vi "HostPC.vi"() -> ()   [LabVIEW 2020]
doc: "Main VI on the host PC. It has an initializisation and an operational phase\n\nThe operational phase has two while loops. One input and one output loop that handle the in/output of the cRio."
uses:
  Status_cRio.ctl
  ElementDTD.lvlib
panel:
  in  "additonal Mass[g]":dbl
  out "Exp_id":i32
  out "Status":T1=enum."1_start_up"
  out "Loginname":string caption="Username"
  in  "OFF":bool
  out "Error PC":bool
  out "SuID":dbl caption="Subject ID" format="%#g"
  out "ImID":dbl caption="Impactor ID" format="%#g"
  in  "Start":bool
  in  "Subject Height[mm]":dbl
  in  "Inspect":bool
  in  "Mode selcection":enum16{"Normal", "Auto", "Manual"}(ring)
  out "Table Position":dbl
  in  "Registerkartenelement":enum32{"Normal", "Auto", "Manual", "Settings"}(tab)
  out "Out of bounds":bool
  in  "Impact Speed [m/s]":dbl
  out "Target Height [mm]":dbl
  in  "Tabel Input [mm]":dbl
  out "Normal Mode:":string
  in  "Table Inputs":dbl[](array[numeric])
  in  "Impact Speeds":dbl[](array[numeric])
  out "Auto Mode:":string
  out "No Data":bool
  out "Index":i32
  in  "Table Input [mm]":dbl
  in  "Carrier Input [mm]":dbl
  in  "Solenoids":bool
  in  "Magnets":bool
  out "Normal/Repair Mode:":string
  in  "Humidity":dbl
  in  "Data Export":bool
  in  "Dialog":bool
  in  "Repair":bool
  in  "Stopp":bool
  out "Name":string
  out "Error cRio":bool
  in  "Skip Cam":bool
  out "Carrier Height":dbl
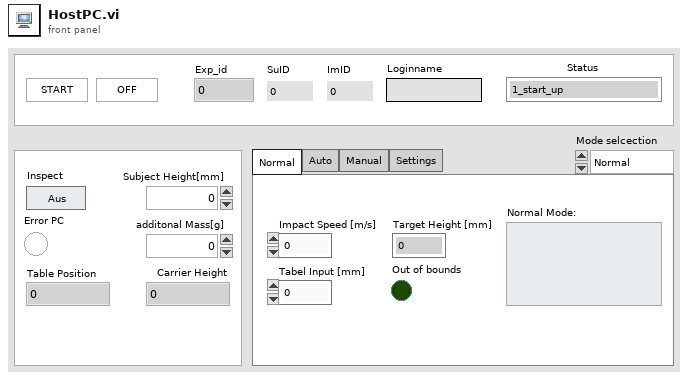
[diagram p1: front panel]
types:
  T1 = typedef "ElementDTD.lvlib/Status_cRio.ctl" = enum16{"0_Error", "1_start_up", "4_moving_to_position", "5_measure", "6_DataExport", "7_turnOff"}
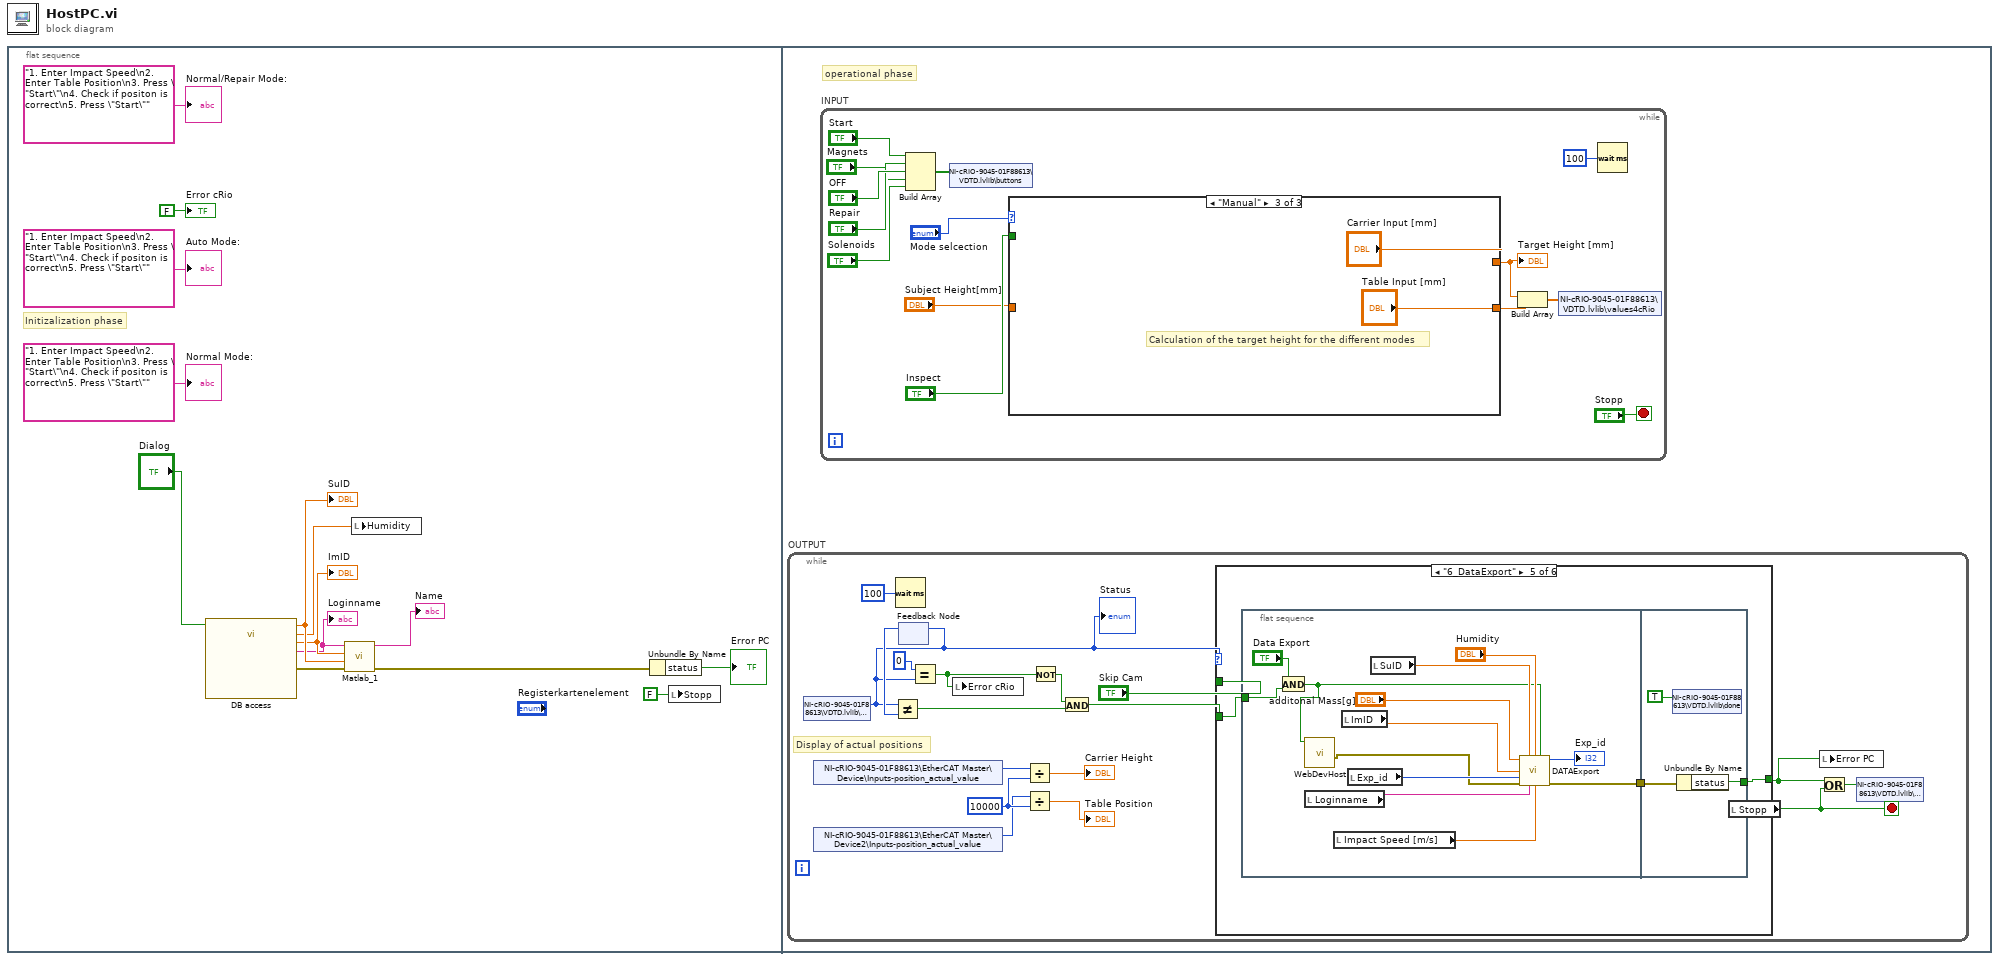
[diagram p0: block diagram]
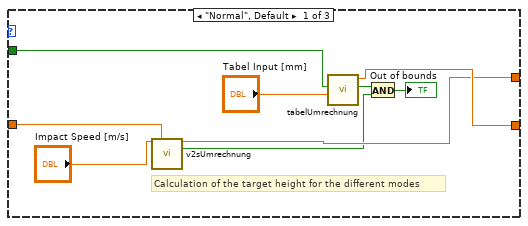
[diagram p2: hidden frame]
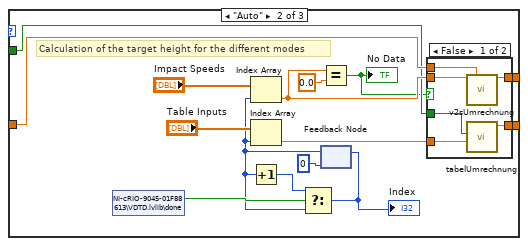
[diagram p3: hidden frame]
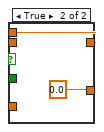
[diagram p4: hidden frame]
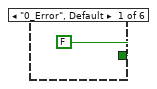
[diagram p5: hidden frame]
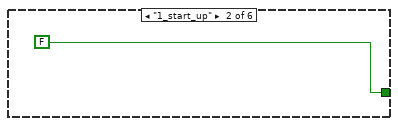
[diagram p6: hidden frame]
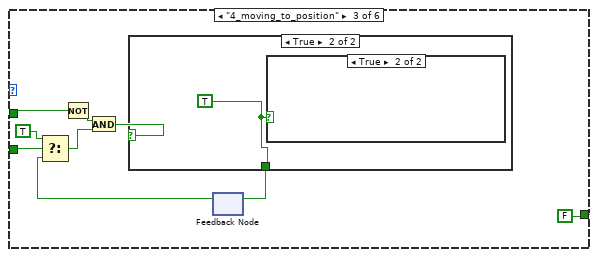
[diagram p7: hidden frame]
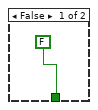
[diagram p8: hidden frame]
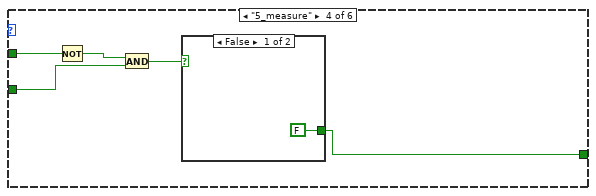
[diagram p10: hidden frame]
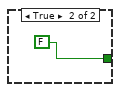
[diagram p11: hidden frame]
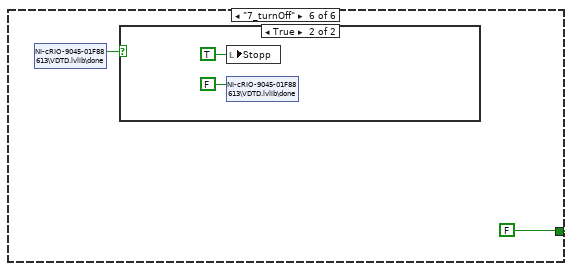
[diagram p12: hidden frame]
diagram:
  n1 = flat-sequence {
    frame #0 {
      # "Initizalization phase"
      n2 = call "DB access"("Enable"="Dialog") -> ("Subject ID"=w14:dbl, "Humidity"=w1:dbl, "Impactor ID"=w13:dbl, "Username"=w12:string, "error out"=w2:errorcluster)  [unwired: 13 in, 1 out]
      "ImID" <- w13
      "SuID" <- w14
      "Loginname" <- w12
      n3 = call "Matlab_1.vi"("Fehler (Eingang, kein Fehler)"=w2, "Subject ID"=w14, "Impactor ID"=w13, "Username"=w12) -> ("Fehler (Ausgang)"=w3:errorcluster, "Name"=→"Name":string)  [unwired: 6 in]
      n4 = local write "Humidity"(w1) -> ()
      n5 = Unbundle By Name(w3) -> ("status"=→"Error PC":bool)
      n6 = local write "Stopp"(FALSE ("Stopp")) -> ()
      "Normal Mode:" <- "1. Enter Impact Speed\n2. Enter Table Position\n3. Press \"Start\"\n4. Check if positon is correct\n5. Press \"Start\"" ("Normal Mode:")
      "Auto Mode:" <- "1. Enter Impact Speed\n2. Enter Table Position\n3. Press \"Start\"\n4. Check if positon is correct\n5. Press \"Start\"" ("Normal Mode:")
      "Error cRio" <- FALSE ("Error cRio")
      "Normal/Repair Mode:" <- "1. Enter Impact Speed\n2. Enter Table Position\n3. Press \"Start\"\n4. Check if positon is correct\n5. Press \"Start\"" ("Normal Mode:")
    }
    frame #1 {
      # "operational phase"
      n7 = while "OUTPUT" {
        stop <- w65 stop-if-true
        w70 = i16 10000 ("y")
        # "Display of actual positions"
        n8 = shared-variable "NI-cRIO-9045-01F88613\\VDTD.lvlib\\state"() -> (w63:T1)  [unwired: 1 in, 1 out]
        "Status" <- w63
        n9 = shared-variable "NI-cRIO-9045-01F88613\\EtherCAT Master\\Device\\Inputs-position_actual_value"() -> (w68:i32)  [unwired: 1 in, 1 out]
        n10 = shared-variable "NI-cRIO-9045-01F88613\\EtherCAT Master\\Device2\\Inputs-position_actual_value"() -> (w69:i32)  [unwired: 1 in, 1 out]
        n11 = Wait (ms)(milliseconds to wait=u32 100 ("Zu wartende ms")) -> ()  [unwired: 1 out]
        n12 = feedback-in #1(w63) -> ()
        n13 = feedback #1() -> (w78:T1)  [unwired: 1 in]
        n14 = Not Equal?(x=w63, y=w78) -> (x != y?=w77:bool)
        n15 = Equal?(x=i16 0, y=w63) -> (x = y?=w72:bool)
        n16 = local write "Error cRio"(w72) -> ()
        n17 = Divide(x=w68, y=w70) -> (x/y=→"Carrier Height":dbl)
        n18 = Divide(x=w69, y=w70) -> (x/y=→"Table Position":dbl)
        n19 = Not(x=w72) -> (.not. x?=w71:bool)
        n20 = And(x=w71, y=w77) -> (x .and. y?=w76:bool)
        n21 = case shown="\"6_DataExport\"" w63 {
          tunnel: [FALSE ("status") FALSE ("status") FALSE ("status") w93 w101 FALSE ("status")] -> w66
          tunnel: w76 -> [_ _ w89 w94 w100 _]
          tunnel: "Skip Cam" -> [_ _ w82 w95 _ _]
          frame "0_Error", Default {
          }
          frame "1_start_up" {
          }
          frame "4_moving_to_position" {
            n22 = Not(x=w82) -> (.not. x?=w85:bool)
            n23 = feedback #2() -> (w90:bool)  [unwired: 1 in]
            n24 = Select(t=TRUE ("s"), s=w89, f=w90) -> (s? t:f=w86:bool)
            n25 = And(x=w85, y=w86) -> (x .and. y?=w87:bool)
            n26 = case shown="True" w87 {
              tunnel: [FALSE w92] -> w84
              frame False {
              }
              frame True {
                w92 = TRUE ("test mode")
                n27 = case shown="True" w92 {
                  frame False {
                  }
                  frame True {
                  }
                }
              }
            }
            n28 = feedback-in #2(w84) -> ()
          }
          frame "5_measure" {
            n29 = Not(x=w95) -> (.not. x?=w96:bool)
            n30 = And(x=w96, y=w94) -> (x .and. y?=w97:bool)
            n31 = case shown="False" w97 {
              tunnel: [FALSE FALSE ("test mode")] -> w93
              frame False {
              }
              frame True {
              }
            }
          }
          frame "6_DataExport" {
            n32 = flat-sequence {
              tunnel: [w109] -> w102
              tunnel: w100 -> [w107]
              tunnel: w102 -> [w118]
              tunnel: [w116] -> w101
              frame #0 {
                n33 = And(x="Data Export", y=w107) -> (x .and. y?=w108:bool)
                n34 = call "WebDevHost.vi"("DataExport"=w108) -> ("error out"=w103:errorcluster)  [unwired: 10 in]
                n35 = local read "Loginname"() -> (w106:string)
                n36 = local read "Impact Speed [m/s]"() -> (w105:dbl)
                n37 = local read "ImID"() -> (w114:dbl)
                n38 = local read "Exp_id"() -> (w111:i32)
                n39 = local read "SuID"() -> (w113:dbl)
                n40 = call "DATAExport.vi"("additonal Mass[g]"="additonal Mass[g]", "Subject ID"=w113, "Humidity"="Humidity", "Data Export"=w108, "Impactor ID"=w114, "Exp_in"=w111, "error in (no error)"=w103, "Username"=w106, "Impact Speed"=w105) -> ("Exp_id"=→"Exp_id":i32, "error out"=w109:errorcluster)  [unwired: 5 in]
              }
              frame #1 {
                n41 = shared-variable "NI-cRIO-9045-01F88613\\VDTD.lvlib\\done"(TRUE ("Done")) -> ()  [unwired: 1 in, 1 out]
                n42 = Unbundle By Name(w118) -> ("status"=w116:bool)
              }
            }
          }
          frame "7_turnOff" {
            n43 = shared-variable "NI-cRIO-9045-01F88613\\VDTD.lvlib\\done"() -> (w120:bool)  [unwired: 1 in, 1 out]
            n44 = case shown="True" w120 {
              frame False {
              }
              frame True {
                n45 = local write "Stopp"(TRUE ("Stopp")) -> ()
                n46 = shared-variable "NI-cRIO-9045-01F88613\\VDTD.lvlib\\done"(FALSE ("Done")) -> ()  [unwired: 1 in, 1 out]
              }
            }
          }
        }
        n47 = local read "Stopp"() -> (w65:bool)
        n48 = local write "Error PC"(w66) -> ()
        n49 = Or(x=w66, y=w65) -> (x .or. y?=w67:bool)
        n50 = shared-variable "NI-cRIO-9045-01F88613\\VDTD.lvlib\\error"(w67) -> ()  [unwired: 1 in, 1 out]
      }
      n51 = while "INPUT" {
        stop <- "Stopp" stop-if-true
        n52 = Build Array("Start", "Repair", "OFF", "Magnets", "Solenoids") -> (w20:bool[])
        n53 = shared-variable "NI-cRIO-9045-01F88613\\VDTD.lvlib\\buttons"(w20) -> ()  [unwired: 1 in, 1 out]
        n54 = case shown="\"Manual\"" "Mode selcection" {
          tunnel: [w34 w47 "Carrier Input [mm]"] -> w23
          tunnel: [w37 w48 "Table Input [mm]"] -> w25
          tunnel: "Inspect" -> [w36 w44 _]
          tunnel: "Subject Height[mm]" -> [w35 w50 _]
          frame "Normal", Default {
            # "Calculation of the target height for the different modes"
            n55 = call "v2sUmrechnung.vi"("Impact Speed [m/s]"="Impact Speed [m/s]", "Test Subject h"=w35) -> ("Hight"=w34:dbl, 6:w31:bool)  [unwired: 12 in]
            n56 = call "tabelUmrechnung.vi"("Tabel Positon"="Tabel Input [mm]", "Inspect"=w36) -> ("In Range?"=w30:bool, "Numerisch"=w37:dbl)  [unwired: 8 in]
            n57 = And(x=w30, y=w31) -> (x .and. y?=→"Out of bounds":bool)
          }
          frame "Auto" {
            # "Calculation of the target height for the different modes"
            n58 = shared-variable "NI-cRIO-9045-01F88613\\VDTD.lvlib\\done"() -> (w41:bool)  [unwired: 1 in, 1 out]
            n59 = feedback #3(0 ("Index")) -> (w39:i32)
            n60 = Index Array(array="Impact Speeds", index=w39) -> (element=w45:dbl)
            n61 = Index Array(array="Table Inputs", index=w39) -> (element=w49:dbl)
            n62 = Increment(x=w39) -> (x+1=w42:i32)
            n63 = Select(t=w42, s=w41, f=w39) -> (s? t:f=w38:i32)
            "Index" <- w38
            n64 = Equal?(x=w45, y=0.0) -> (x = y?=w43:bool)
            "No Data" <- w43
            n65 = feedback-in #3(w38) -> ()
            n66 = case shown="False" w43 {
              tunnel: w50 -> [w58 w59]
              tunnel: w45 -> [w57 _]
              tunnel: w49 -> [w56 _]
              tunnel: w44 -> [w55 _]
              tunnel: [w54 0.0 ("Numerisch")] -> w48
              tunnel: [w53 w59] -> w47
              frame False {
                n67 = call "v2sUmrechnung.vi"("Impact Speed [m/s]"=w57, "Test Subject h"=w58) -> ("Hight"=w53:dbl)  [unwired: 12 in, 1 out]
                n68 = call "tabelUmrechnung.vi"("Tabel Positon"=w56, "Inspect"=w55) -> ("Numerisch"=w54:dbl)  [unwired: 8 in, 1 out]
              }
              frame True {
              }
            }
          }
          frame "Manual" {
            # "Calculation of the target height for the different modes"
          }
        }
        "Target Height [mm]" <- w23
        n69 = Build Array(w23, w25) -> (w27:dbl[])
        n70 = shared-variable "NI-cRIO-9045-01F88613\\VDTD.lvlib\\values4cRio"(w27) -> ()  [unwired: 1 in, 1 out]
        n71 = Wait (ms)(milliseconds to wait=u32 100 ("Zu wartende ms")) -> ()  [unwired: 1 out]
      }
    }
  }
